vi "反控参数设置.vi"(8 "value time":timestamp, 9 "value float":sgl, 10 "设置参数":T2(ring)=enum."CODMn", 11 "设置类型":T1(ring)=enum."i13002") -> ()   [LabVIEW 2016, in "MB SLAVE.lvlib"]
uses:
  MB SLAVE.lvlib
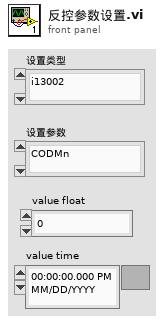
[diagram p1: front panel]
types:
  T1 = enum16{"i13001", "i13002", "i13003", "i13004", "i13005", "i13006", "i13007", "i13008", "i13009", "i13010", "i13011", "i13012", "i13013", "i13014", "i13015", "i13016", "i13017", "i13101", "i13102", "i13103", "i13104", "i13105", "i13106", "i13107", "i13108", "i13109", "i13110"}
  T2 = enum16{"", "CODMn", "PH", "氨氮", "总氮", "总磷", "CODCr", "电导率", "水温", "溶解氧", "浊度", "叶绿素", "藻密度", "ORP"}
  T3 = cluster{"status":bool, "代码":u16, "source":string}
  T4 = typedef "CODMn交互.ctl" = cluster{"COD浓度（mg/L)":dbl, "水样启动时间":timestamp, "加标回收启动时间":timestamp, "CODMn工作状态":enum16{"空闲", "水样测试", "标样核查", "零点核查", "跨度核查", "空白测试", "平行样测试", "加标回收", "空白校准", "标样校准", "初始化（清洗）"}, "多列列表框":i32, "平台试剂余量百分比":sgl, "关键参数":cluster{"测量量程":dbl, "测量精度":dbl, "测量间隔":dbl, "消解温度":dbl, "消解时长":dbl, "空白校准时间":timestamp, "曲线截距":dbl, "曲线斜率":dbl, "测量检出限":dbl, "测量信号值":dbl, "线性相关系数":dbl, "二次多项式系数":dbl, "标样校准时间":timestamp, "稀释倍数":dbl, "三项式系数":dbl, "空白标定系数":dbl, "量程系数":dbl, "F0/ORPA":dbl, "F1/ORPB":dbl, "F2/ORPK":dbl, "F3":dbl, "F4":dbl, "F5":dbl, "F6":dbl, "F7":dbl, "X0/滴定数":dbl, "量程":dbl}, "关键参数改变":bool, "校准信息":cluster{"低标液1浓度":dbl, "低标液1信号值":dbl, "低标液1启用":u16, "低标液2浓度":dbl, "低标液2信号值":dbl, "低标液2启用":u16, "低标液3浓度":dbl, "低标液3信号值":dbl, "低标液3启用":u16, "低标液4浓度":dbl, "低标液4信号值":dbl, "低标液4启用":u16, "低标液5浓度":dbl, "低标液5信号值":dbl, "低标液5启用":u16, "高标液1浓度":dbl, "高标液1信号值":dbl, "高标液1启用":u16, "高标液2浓度":dbl, "高标液2信号值":dbl, "高标液2启用":u16, "高标液3浓度":dbl, "高标液3信号值":dbl, "高标液3启用":u16, "高标液4浓度":dbl, "高标液4信号值":dbl, "高标液4启用":u16, "高标液5浓度":dbl, "高标液5信号值":dbl, "高标液5启用":u16}, "校准信息改变":bool}
  T5 = cluster{"测量量程":dbl, "测量精度":dbl, "测量间隔":dbl, "消解温度":dbl, "消解时长":dbl, "空白校准时间":timestamp, "曲线截距":dbl, "曲线斜率":dbl, "测量检出限":dbl, "测量信号值":dbl, "线性相关系数":dbl, "二次多项式系数":dbl, "标样校准时间":timestamp, "稀释倍数":dbl, "三项式系数":dbl, "空白标定系数":dbl, "量程系数":dbl, "F0/ORPA":dbl, "F1/ORPB":dbl, "F2/ORPK":dbl, "F3":dbl, "F4":dbl, "F5":dbl, "F6":dbl, "F7":dbl, "X0/滴定数":dbl, "量程":dbl}
  T6 = typedef "氨氮交互.ctl" = cluster{"状态告警区":cluster{"系统时间":timestamp, "工作状态":u16, "测量模式":enum16{"待机", "连续模式", "周期模式", "定点模式", "受控模式", "手动模式"}, "告警代码":u16, "故障代码":u16, "日志代码":u16, "软件版本":u16, "F0":sgl, "F1":sgl, "F2":sgl, "F3":sgl, "T":sgl, "H":sgl, "id":u16, "flowid":u16, "量程":u16, "总磷控温温度1":sgl, "营养盐控温温度2":sgl, "ADC":sgl}, "平台试剂余量百分比":sgl, "关键参数":cluster{"测量量程":dbl, "测量精度":dbl, "测量间隔":dbl, "消解温度":dbl, "消解时长":dbl, "空白校准时间":timestamp, "曲线截距":dbl, "曲线斜率":dbl, "测量检出限":dbl, "测量信号值":dbl, "线性相关系数":dbl, "二次多项式系数":dbl, "标样校准时间":timestamp, "稀释倍数":dbl, "三项式系数":dbl, "空白标定系数":dbl, "量程系数":dbl, "F0/ORPA":dbl, "F1/ORPB":dbl, "F2/ORPK":dbl, "F3":dbl, "F4":dbl, "F5":dbl, "F6":dbl, "F7":dbl, "X0/滴定数":dbl, "量程":dbl}, "关键参数改变":bool, "校准信息":cluster{"低标液1浓度":dbl, "低标液1信号值":dbl, "低标液1启用":u16, "低标液2浓度":dbl, "低标液2信号值":dbl, "低标液2启用":u16, "低标液3浓度":dbl, "低标液3信号值":dbl, "低标液3启用":u16, "低标液4浓度":dbl, "低标液4信号值":dbl, "低标液4启用":u16, "低标液5浓度":dbl, "低标液5信号值":dbl, "低标液5启用":u16, "高标液1浓度":dbl, "高标液1信号值":dbl, "高标液1启用":u16, "高标液2浓度":dbl, "高标液2信号值":dbl, "高标液2启用":u16, "高标液3浓度":dbl, "高标液3信号值":dbl, "高标液3启用":u16, "高标液4浓度":dbl, "高标液4信号值":dbl, "高标液4启用":u16, "高标液5浓度":dbl, "高标液5信号值":dbl, "高标液5启用":u16}, "校准信息改变":bool}
  T7 = typedef "总氮交互.ctl" = cluster{"状态告警区":cluster{"系统时间":timestamp, "工作状态":u16, "测量模式":enum16{"待机", "连续模式", "周期模式", "定点模式", "受控模式", "手动模式"}, "告警代码":u16, "故障代码":u16, "日志代码":u16, "软件版本":u16, "F0":sgl, "F1":sgl, "F2":sgl, "F3":sgl, "T":sgl, "H":sgl, "id":u16, "flowid":u16, "量程":u16, "总磷控温温度1":sgl, "营养盐控温温度2":sgl, "ADC":sgl}, "平台试剂余量百分比":sgl, "关键参数":cluster{"测量量程":dbl, "测量精度":dbl, "测量间隔":dbl, "消解温度":dbl, "消解时长":dbl, "空白校准时间":timestamp, "曲线截距":dbl, "曲线斜率":dbl, "测量检出限":dbl, "测量信号值":dbl, "线性相关系数":dbl, "二次多项式系数":dbl, "标样校准时间":timestamp, "稀释倍数":dbl, "三项式系数":dbl, "空白标定系数":dbl, "量程系数":dbl, "F0/ORPA":dbl, "F1/ORPB":dbl, "F2/ORPK":dbl, "F3":dbl, "F4":dbl, "F5":dbl, "F6":dbl, "F7":dbl, "X0/滴定数":dbl, "量程":dbl}, "关键参数改变":bool, "校准信息":cluster{"低标液1浓度":dbl, "低标液1信号值":dbl, "低标液1启用":u16, "低标液2浓度":dbl, "低标液2信号值":dbl, "低标液2启用":u16, "低标液3浓度":dbl, "低标液3信号值":dbl, "低标液3启用":u16, "低标液4浓度":dbl, "低标液4信号值":dbl, "低标液4启用":u16, "低标液5浓度":dbl, "低标液5信号值":dbl, "低标液5启用":u16, "高标液1浓度":dbl, "高标液1信号值":dbl, "高标液1启用":u16, "高标液2浓度":dbl, "高标液2信号值":dbl, "高标液2启用":u16, "高标液3浓度":dbl, "高标液3信号值":dbl, "高标液3启用":u16, "高标液4浓度":dbl, "高标液4信号值":dbl, "高标液4启用":u16, "高标液5浓度":dbl, "高标液5信号值":dbl, "高标液5启用":u16}, "校准信息改变":bool}
  T8 = typedef "总磷交互.ctl" = cluster{"状态告警区":cluster{"系统时间":timestamp, "工作状态":u16, "测量模式":enum16{"待机", "连续模式", "周期模式", "定点模式", "受控模式", "手动模式"}, "告警代码":u16, "故障代码":u16, "日志代码":u16, "软件版本":u16, "F0":sgl, "F1":sgl, "F2":sgl, "F3":sgl, "T":sgl, "H":sgl, "id":u16, "flowid":u16, "量程":u16, "总磷控温温度1":sgl, "营养盐控温温度2":sgl, "ADC":sgl}, "平台试剂余量百分比":sgl, "关键参数":cluster{"测量量程":dbl, "测量精度":dbl, "测量间隔":dbl, "消解温度":dbl, "消解时长":dbl, "空白校准时间":timestamp, "曲线截距":dbl, "曲线斜率":dbl, "测量检出限":dbl, "测量信号值":dbl, "线性相关系数":dbl, "二次多项式系数":dbl, "标样校准时间":timestamp, "稀释倍数":dbl, "三项式系数":dbl, "空白标定系数":dbl, "量程系数":dbl, "F0/ORPA":dbl, "F1/ORPB":dbl, "F2/ORPK":dbl, "F3":dbl, "F4":dbl, "F5":dbl, "F6":dbl, "F7":dbl, "X0/滴定数":dbl, "量程":dbl}, "关键参数改变":bool, "校准信息":cluster{"低标液1浓度":dbl, "低标液1信号值":dbl, "低标液1启用":u16, "低标液2浓度":dbl, "低标液2信号值":dbl, "低标液2启用":u16, "低标液3浓度":dbl, "低标液3信号值":dbl, "低标液3启用":u16, "低标液4浓度":dbl, "低标液4信号值":dbl, "低标液4启用":u16, "低标液5浓度":dbl, "低标液5信号值":dbl, "低标液5启用":u16, "高标液1浓度":dbl, "高标液1信号值":dbl, "高标液1启用":u16, "高标液2浓度":dbl, "高标液2信号值":dbl, "高标液2启用":u16, "高标液3浓度":dbl, "高标液3信号值":dbl, "高标液3启用":u16, "高标液4浓度":dbl, "高标液4信号值":dbl, "高标液4启用":u16, "高标液5浓度":dbl, "高标液5信号值":dbl, "高标液5启用":u16}, "校准信息改变":bool}
  T9 = typedef "CODCr交互.ctl" = cluster{"状态告警区":cluster{"系统时间":timestamp, "工作状态":u16, "测量模式":enum16{"待机", "连续模式", "周期模式", "定点模式", "受控模式", "手动模式"}, "告警代码":u16, "故障代码":u16, "日志代码":u16, "软件版本":u16, "F0":sgl, "F1":sgl, "F2":sgl, "F3":sgl, "T":sgl, "H":sgl, "id":u16, "flowid":u16, "量程":u16, "总磷控温温度1":sgl, "营养盐控温温度2":sgl, "ADC":sgl}, "平台试剂余量百分比":sgl, "关键参数":cluster{"测量量程":dbl, "测量精度":dbl, "测量间隔":dbl, "消解温度":dbl, "消解时长":dbl, "空白校准时间":timestamp, "曲线截距":dbl, "曲线斜率":dbl, "测量检出限":dbl, "测量信号值":dbl, "线性相关系数":dbl, "二次多项式系数":dbl, "标样校准时间":timestamp, "稀释倍数":dbl, "三项式系数":dbl, "空白标定系数":dbl, "量程系数":dbl, "F0/ORPA":dbl, "F1/ORPB":dbl, "F2/ORPK":dbl, "F3":dbl, "F4":dbl, "F5":dbl, "F6":dbl, "F7":dbl, "X0/滴定数":dbl, "量程":dbl}, "关键参数改变":bool, "校准信息":cluster{"低标液1浓度":dbl, "低标液1信号值":dbl, "低标液1启用":u16, "低标液2浓度":dbl, "低标液2信号值":dbl, "低标液2启用":u16, "低标液3浓度":dbl, "低标液3信号值":dbl, "低标液3启用":u16, "低标液4浓度":dbl, "低标液4信号值":dbl, "低标液4启用":u16, "低标液5浓度":dbl, "低标液5信号值":dbl, "低标液5启用":u16, "高标液1浓度":dbl, "高标液1信号值":dbl, "高标液1启用":u16, "高标液2浓度":dbl, "高标液2信号值":dbl, "高标液2启用":u16, "高标液3浓度":dbl, "高标液3信号值":dbl, "高标液3启用":u16, "高标液4浓度":dbl, "高标液4信号值":dbl, "高标液4启用":u16, "高标液5浓度":dbl, "高标液5信号值":dbl, "高标液5启用":u16}, "校准信息改变":bool}
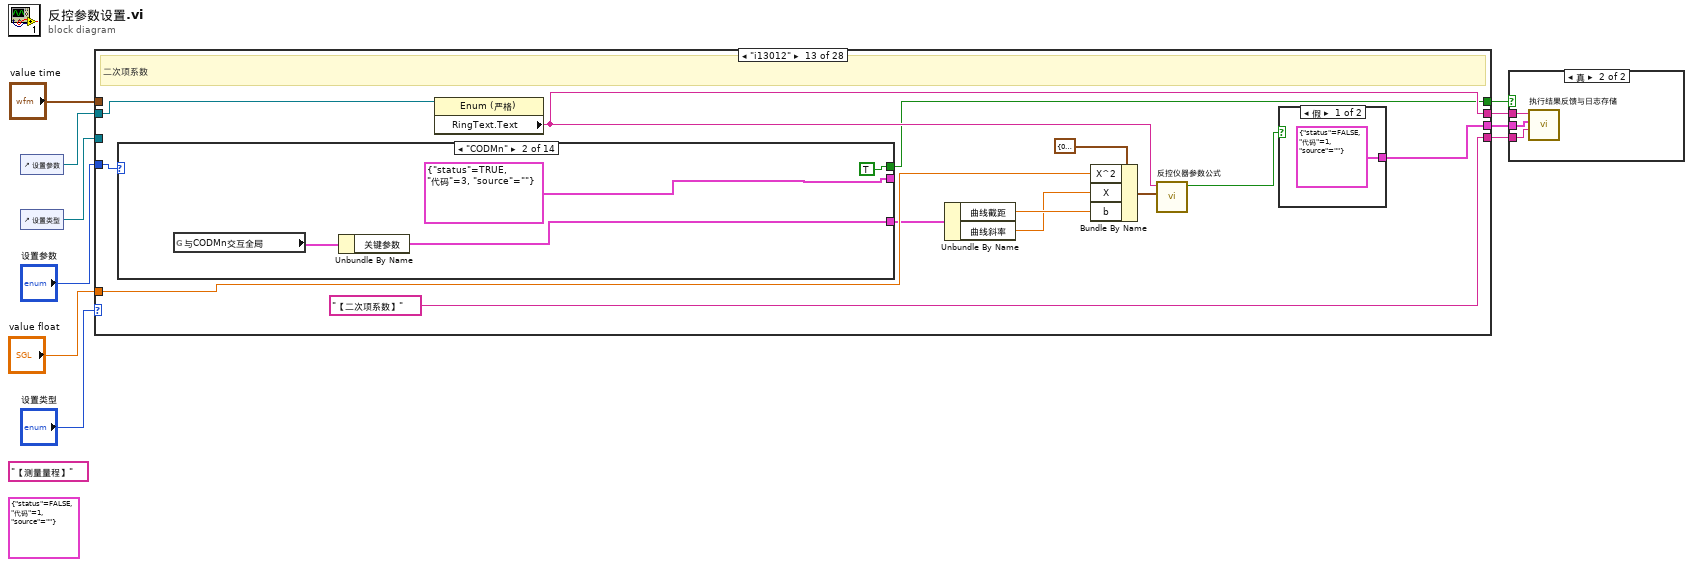
[diagram p0: block diagram]
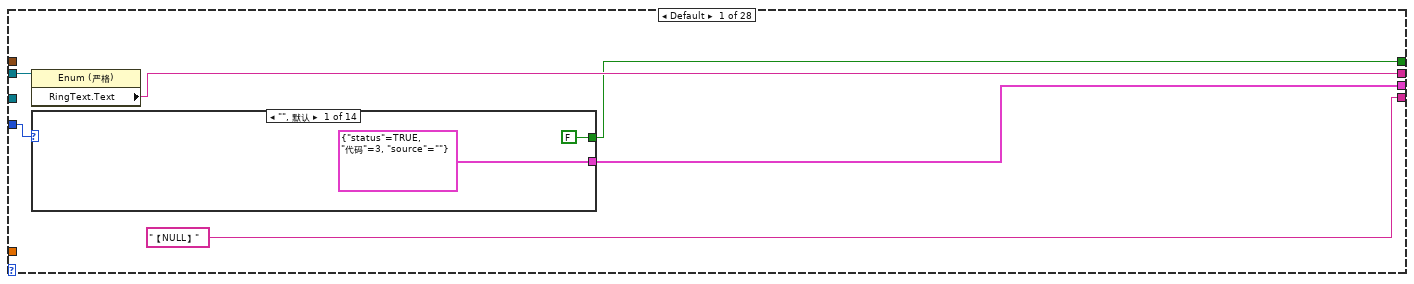
[diagram p3: hidden frame]
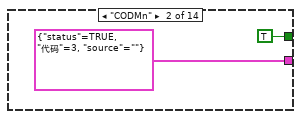
[diagram p4: hidden frame]
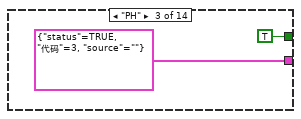
[diagram p5: hidden frame]
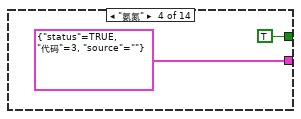
[diagram p6: hidden frame]
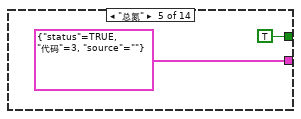
[diagram p7: hidden frame]
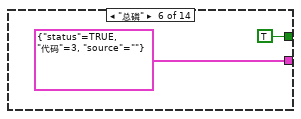
[diagram p8: hidden frame]
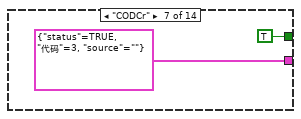
[diagram p9: hidden frame]
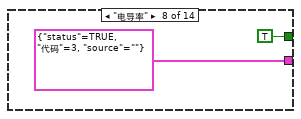
[diagram p10: hidden frame]
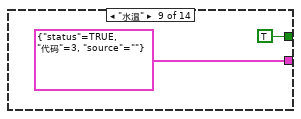
[diagram p11: hidden frame]
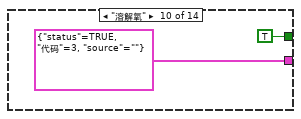
[diagram p12: hidden frame]
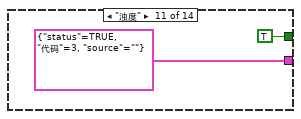
[diagram p13: hidden frame]
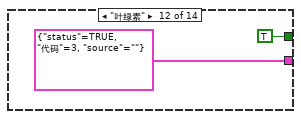
[diagram p14: hidden frame]
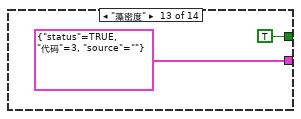
[diagram p15: hidden frame]
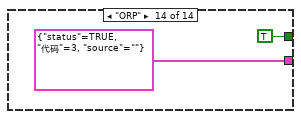
[diagram p16: hidden frame]
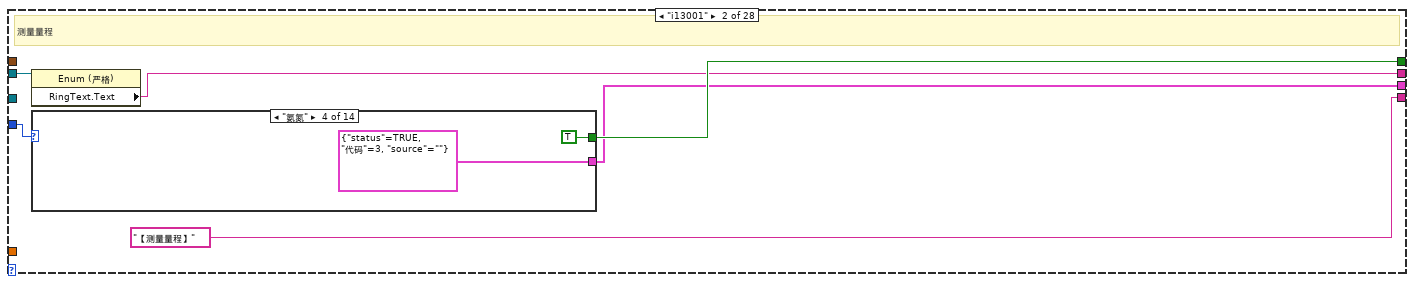
[diagram p17: hidden frame]
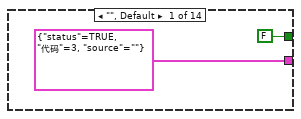
[diagram p18: hidden frame]
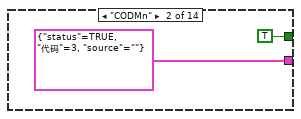
[diagram p19: hidden frame]
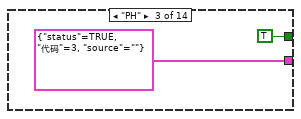
[diagram p20: hidden frame]
diagram:
  (unwired) T3 {"status"=FALSE, "代码"=1, "source"=""} ("error out")
  (unwired) "【测量量程】" ("日志信息")
  n1 = control-ref of="设置参数"() -> (w7:refnum<vi>)
  n2 = control-ref of="设置类型"() -> (w1:refnum<vi>)
  n3 = case shown="\"i13012\"" "设置类型" {
    tunnel: "设置参数" -> [w16 w50 w83 w114 w150 w193 w233 w269 w329 w373 w408 w444 w477 w528 w562 w596 w630 w664 w698 w732 w766 w804 w834 w868 w902 w936 w970 w1004]
    tunnel: [w12 w49 w80 w116 w152 w196 w236 w268 w332 w376 w410 w442 w476 w531 w565 w599 w633 w667 w701 w735 w769 w801 w837 w871 w905 w939 w973 w1007] -> w8
    tunnel: w7 -> [w15 w46 w84 w113 w154 w194 w234 w278 w330 w374 w407 w445 w486 w529 w563 w597 w631 w665 w699 w733 w767 w805 w835 w869 w903 w937 w971 w1005]
    tunnel: [w14 w45 w82 w118 w149 w190 w238 w274 w323 w378 w412 w446 w480 w533 w567 w601 w635 w669 w703 w737 w771 w803 w839 w873 w907 w941 w975 w1009] -> w6
    tunnel: ["【NULL】" ("日志信息") "【测量量程】" ("日志信息") "【测量精度】" ("日志信息") "【测量间隔】" ("日志信息") "【消解温度】" ("日志信息") "【消解时间】" ("日志信息") "【空白校准时间】" ("日志信息") "【曲线截距】" ("日志信息") "【曲线斜率】" ("日志信息") "【测量检出限】" ("日志信息") "【测量信号值】" ("日志信息") "【线性相关系数】" ("日志信息") "【二次项系数】" ("日志信息") "【标样校准时间】" ("日志信息") "【稀释倍数】" ("日志信息") "【三项式系数】" ("日志信息") "【空白标定系数】" ("日志信息") "【量程系数】" ("日志信息") "【F0/ORPA】" ("日志信息") "【F1/ORPB】" ("日志信息") "【F2/ORPK】" ("日志信息") "【F3】" ("日志信息") "【F4】" ("日志信息") "【F5】" ("日志信息") "【F6】" ("日志信息") "【F7】" ("日志信息") "【X0/滴定数】" ("日志信息") "【量程】" ("日志信息")] -> w5
    tunnel: [w13 w47 w81 w117 w153 w197 w237 w272 w325 w377 w411 w443 w482 w532 w566 w600 w634 w668 w702 w736 w770 w802 w838 w872 w906 w940 w974 w1008] -> w4
    tunnel: "value float" -> [_ _ _ _ w148 w192 _ w275 w324 _ _ _ w481 _ _ _ _ _ _ _ _ _ _ _ _ _ _ _]
    tunnel: "value time" -> [_ _ _ _ _ _ _ _ _ _ _ _ _ _ _ _ _ _ _ _ _ _ _ _ _ _ _ _]
    tunnel: w1 -> [_ _ _ _ w147 w191 _ _ _ _ _ _ _ _ _ _ _ _ _ _ _ _ _ _ _ _ _ _]
    frame Default {
      n4 = property class="Enum (严格)"(reference=w15) -> ("RingText.Text"=w14:string)  [unwired: 1 in, 2 out]
      n5 = case shown="\"\", 默认" w16 {
        tunnel: [FALSE TRUE TRUE TRUE TRUE TRUE TRUE TRUE TRUE TRUE TRUE TRUE TRUE TRUE] -> w12
        tunnel: [T3 {"status"=TRUE, "代码"=3, "source"=""} ("error out") T3 {"status"=TRUE, "代码"=3, "source"=""} ("error out") T3 {"status"=TRUE, "代码"=3, "source"=""} ("error out") T3 {"status"=TRUE, "代码"=3, "source"=""} ("error out") T3 {"status"=TRUE, "代码"=3, "source"=""} ("error out") T3 {"status"=TRUE, "代码"=3, "source"=""} ("error out") T3 {"status"=TRUE, "代码"=3, "source"=""} ("error out") T3 {"status"=TRUE, "代码"=3, "source"=""} ("error out") T3 {"status"=TRUE, "代码"=3, "source"=""} ("error out") T3 {"status"=TRUE, "代码"=3, "source"=""} ("error out") T3 {"status"=TRUE, "代码"=3, "source"=""} ("error out") T3 {"status"=TRUE, "代码"=3, "source"=""} ("error out") T3 {"status"=TRUE, "代码"=3, "source"=""} ("error out") T3 {"status"=TRUE, "代码"=3, "source"=""} ("error out")] -> w13
        frame "", Default {
        }
        frame "CODMn" {
        }
        frame "PH" {
        }
        frame "氨氮" {
        }
        frame "总氮" {
        }
        frame "总磷" {
        }
        frame "CODCr" {
        }
        frame "电导率" {
        }
        frame "水温" {
        }
        frame "溶解氧" {
        }
        frame "浊度" {
        }
        frame "叶绿素" {
        }
        frame "藻密度" {
        }
        frame "ORP" {
        }
      }
    }
    frame "i13001" {
      # "测量量程"
      n6 = property class="Enum (严格)"(reference=w46) -> ("RingText.Text"=w45:string)  [unwired: 1 in, 2 out]
      n7 = case shown="\"氨氮\"" w50 {
        tunnel: [FALSE TRUE TRUE TRUE TRUE TRUE TRUE TRUE TRUE TRUE TRUE TRUE TRUE TRUE] -> w49
        tunnel: [T3 {"status"=TRUE, "代码"=3, "source"=""} ("error out") T3 {"status"=TRUE, "代码"=3, "source"=""} ("error out") T3 {"status"=TRUE, "代码"=3, "source"=""} ("error out") T3 {"status"=TRUE, "代码"=3, "source"=""} ("error out") T3 {"status"=TRUE, "代码"=3, "source"=""} ("error out") T3 {"status"=TRUE, "代码"=3, "source"=""} ("error out") T3 {"status"=TRUE, "代码"=3, "source"=""} ("error out") T3 {"status"=TRUE, "代码"=3, "source"=""} ("error out") T3 {"status"=TRUE, "代码"=3, "source"=""} ("error out") T3 {"status"=TRUE, "代码"=3, "source"=""} ("error out") T3 {"status"=TRUE, "代码"=3, "source"=""} ("error out") T3 {"status"=TRUE, "代码"=3, "source"=""} ("error out") T3 {"status"=TRUE, "代码"=3, "source"=""} ("error out") T3 {"status"=TRUE, "代码"=3, "source"=""} ("error out")] -> w47
        frame "", Default {
        }
        frame "CODMn" {
        }
        frame "PH" {
        }
        frame "氨氮" {
        }
        frame "总氮" {
        }
        frame "总磷" {
        }
        frame "CODCr" {
        }
        frame "电导率" {
        }
        frame "水温" {
        }
        frame "溶解氧" {
        }
        frame "浊度" {
        }
        frame "叶绿素" {
        }
        frame "藻密度" {
        }
        frame "ORP" {
        }
      }
    }
    frame "i13002" {
      # "测量精度"
      n8 = property class="Enum (严格)"(reference=w84) -> ("RingText.Text"=w82:string)  [unwired: 1 in, 2 out]
      n9 = case shown="\"CODMn\"" w83 {
        tunnel: [FALSE TRUE TRUE TRUE TRUE TRUE TRUE TRUE TRUE TRUE TRUE TRUE TRUE TRUE] -> w80
        tunnel: [T3 {"status"=TRUE, "代码"=3, "source"=""} ("error out") T3 {"status"=TRUE, "代码"=3, "source"=""} ("error out") T3 {"status"=TRUE, "代码"=3, "source"=""} ("error out") T3 {"status"=TRUE, "代码"=3, "source"=""} ("error out") T3 {"status"=TRUE, "代码"=3, "source"=""} ("error out") T3 {"status"=TRUE, "代码"=3, "source"=""} ("error out") T3 {"status"=TRUE, "代码"=3, "source"=""} ("error out") T3 {"status"=TRUE, "代码"=3, "source"=""} ("error out") T3 {"status"=TRUE, "代码"=3, "source"=""} ("error out") T3 {"status"=TRUE, "代码"=3, "source"=""} ("error out") T3 {"status"=TRUE, "代码"=3, "source"=""} ("error out") T3 {"status"=TRUE, "代码"=3, "source"=""} ("error out") T3 {"status"=TRUE, "代码"=3, "source"=""} ("error out") T3 {"status"=TRUE, "代码"=3, "source"=""} ("error out")] -> w81
        frame "", Default {
        }
        frame "CODMn" {
        }
        frame "PH" {
        }
        frame "氨氮" {
        }
        frame "总氮" {
        }
        frame "总磷" {
        }
        frame "CODCr" {
        }
        frame "电导率" {
        }
        frame "水温" {
        }
        frame "溶解氧" {
        }
        frame "浊度" {
        }
        frame "叶绿素" {
        }
        frame "藻密度" {
        }
        frame "ORP" {
        }
      }
    }
    frame "i13003" {
      # "测量间隔"
      n10 = property class="Enum (严格)"(reference=w113) -> ("RingText.Text"=w118:string)  [unwired: 1 in, 2 out]
      n11 = case shown="\"CODMn\"" w114 {
        tunnel: [FALSE TRUE TRUE TRUE TRUE TRUE TRUE TRUE TRUE TRUE TRUE TRUE TRUE TRUE] -> w116
        tunnel: [T3 {"status"=TRUE, "代码"=3, "source"=""} ("error out") T3 {"status"=TRUE, "代码"=3, "source"=""} ("error out") T3 {"status"=TRUE, "代码"=3, "source"=""} ("error out") T3 {"status"=TRUE, "代码"=3, "source"=""} ("error out") T3 {"status"=TRUE, "代码"=3, "source"=""} ("error out") T3 {"status"=TRUE, "代码"=3, "source"=""} ("error out") T3 {"status"=TRUE, "代码"=3, "source"=""} ("error out") T3 {"status"=TRUE, "代码"=3, "source"=""} ("error out") T3 {"status"=TRUE, "代码"=3, "source"=""} ("error out") T3 {"status"=TRUE, "代码"=3, "source"=""} ("error out") T3 {"status"=TRUE, "代码"=3, "source"=""} ("error out") T3 {"status"=TRUE, "代码"=3, "source"=""} ("error out") T3 {"status"=TRUE, "代码"=3, "source"=""} ("error out") T3 {"status"=TRUE, "代码"=3, "source"=""} ("error out")] -> w117
        frame "", Default {
        }
        frame "CODMn" {
        }
        frame "PH" {
        }
        frame "氨氮" {
        }
        frame "总氮" {
        }
        frame "总磷" {
        }
        frame "CODCr" {
        }
        frame "电导率" {
        }
        frame "水温" {
        }
        frame "溶解氧" {
        }
        frame "浊度" {
        }
        frame "叶绿素" {
        }
        frame "藻密度" {
        }
        frame "ORP" {
        }
      }
    }
    frame "i13004" {
      # "消解温度"
      n12 = property class="Enum (严格)"(reference=w154) -> ("RingText.Text"=w149:string)  [unwired: 1 in, 2 out]
      n13 = case shown="\"氨氮\"" w150 {
        tunnel: [FALSE TRUE TRUE TRUE TRUE TRUE TRUE TRUE TRUE TRUE TRUE TRUE TRUE TRUE] -> w152
        tunnel: [T3 {"status"=TRUE, "代码"=3, "source"=""} ("error out") w159 T3 {"status"=TRUE, "代码"=3, "source"=""} ("error out") T3 {"status"=TRUE, "代码"=3, "source"=""} ("error out") T3 {"status"=TRUE, "代码"=3, "source"=""} ("error out") T3 {"status"=TRUE, "代码"=3, "source"=""} ("error out") T3 {"status"=TRUE, "代码"=3, "source"=""} ("error out") T3 {"status"=TRUE, "代码"=3, "source"=""} ("error out") T3 {"status"=TRUE, "代码"=3, "source"=""} ("error out") T3 {"status"=TRUE, "代码"=3, "source"=""} ("error out") T3 {"status"=TRUE, "代码"=3, "source"=""} ("error out") T3 {"status"=TRUE, "代码"=3, "source"=""} ("error out") T3 {"status"=TRUE, "代码"=3, "source"=""} ("error out") T3 {"status"=TRUE, "代码"=3, "source"=""} ("error out")] -> w153
        tunnel: w149 -> [_ w162 _ _ _ _ _ _ _ _ _ _ _ _]
        tunnel: w148 -> [_ w161 _ _ _ _ _ _ _ _ _ _ _ _]
        tunnel: w147 -> [_ w158 _ _ _ _ _ _ _ _ _ _ _ _]
        frame "", Default {
        }
        frame "CODMn" {
          n14 = property class="Enum (严格)"(reference=w158) -> ("RingText.Text"=w157:string)  [unwired: 1 in, 2 out]
          n15 = call "反控仪器单参数通用.vi"("参数"=w162, "value float"=w161, "chose"=w157) -> ("超时？"=w160:bool)  [unwired: 7 in, 1 out]
          n16 = case shown="假" w160 {
            tunnel: [T3 {"status"=FALSE, "代码"=1, "source"=""} ("error out") T3 {"status"=TRUE, "代码"=4, "source"=""} ("error out")] -> w159
            frame False {
            }
            frame True {
            }
          }
        }
        frame "PH" {
        }
        frame "氨氮" {
        }
        frame "总氮" {
        }
        frame "总磷" {
        }
        frame "CODCr" {
        }
        frame "电导率" {
        }
        frame "水温" {
        }
        frame "溶解氧" {
        }
        frame "浊度" {
        }
        frame "叶绿素" {
        }
        frame "藻密度" {
        }
        frame "ORP" {
        }
      }
    }
    frame "i13005" {
      # "消解时间"
      n17 = property class="Enum (严格)"(reference=w194) -> ("RingText.Text"=w190:string)  [unwired: 1 in, 2 out]
      n18 = case shown="\"CODMn\"" w193 {
        tunnel: [FALSE TRUE TRUE TRUE TRUE TRUE TRUE TRUE TRUE TRUE TRUE TRUE TRUE TRUE] -> w196
        tunnel: [T3 {"status"=TRUE, "代码"=3, "source"=""} ("error out") w200 T3 {"status"=TRUE, "代码"=3, "source"=""} ("error out") T3 {"status"=TRUE, "代码"=3, "source"=""} ("error out") T3 {"status"=TRUE, "代码"=3, "source"=""} ("error out") T3 {"status"=TRUE, "代码"=3, "source"=""} ("error out") T3 {"status"=TRUE, "代码"=3, "source"=""} ("error out") T3 {"status"=TRUE, "代码"=3, "source"=""} ("error out") T3 {"status"=TRUE, "代码"=3, "source"=""} ("error out") T3 {"status"=TRUE, "代码"=3, "source"=""} ("error out") T3 {"status"=TRUE, "代码"=3, "source"=""} ("error out") T3 {"status"=TRUE, "代码"=3, "source"=""} ("error out") T3 {"status"=TRUE, "代码"=3, "source"=""} ("error out") T3 {"status"=TRUE, "代码"=3, "source"=""} ("error out")] -> w197
        tunnel: w192 -> [_ w203 _ _ _ _ _ _ _ _ _ _ _ _]
        tunnel: w191 -> [_ w202 _ _ _ _ _ _ _ _ _ _ _ _]
        tunnel: w190 -> [_ w201 _ _ _ _ _ _ _ _ _ _ _ _]
        frame "", Default {
        }
        frame "CODMn" {
          n19 = property class="Enum (严格)"(reference=w202) -> ("RingText.Text"=w204:string)  [unwired: 1 in, 2 out]
          n20 = call "反控仪器单参数通用.vi"("参数"=w201, "value float"=w203, "chose"=w204) -> ("超时？"=w205:bool)  [unwired: 7 in, 1 out]
          n21 = case shown="假" w205 {
            tunnel: [T3 {"status"=FALSE, "代码"=1, "source"=""} ("error out") T3 {"status"=TRUE, "代码"=4, "source"=""} ("error out")] -> w200
            frame False {
            }
            frame True {
            }
          }
        }
        frame "PH" {
        }
        frame "氨氮" {
        }
        frame "总氮" {
        }
        frame "总磷" {
        }
        frame "CODCr" {
        }
        frame "电导率" {
        }
        frame "水温" {
        }
        frame "溶解氧" {
        }
        frame "浊度" {
        }
        frame "叶绿素" {
        }
        frame "藻密度" {
        }
        frame "ORP" {
        }
      }
    }
    frame "i13006" {
      # "空白校准时间"
      n22 = property class="Enum (严格)"(reference=w234) -> ("RingText.Text"=w238:string)  [unwired: 1 in, 2 out]
      n23 = case shown="\"CODMn\"" w233 {
        tunnel: [FALSE TRUE TRUE TRUE TRUE TRUE TRUE TRUE TRUE TRUE TRUE TRUE TRUE TRUE] -> w236
        tunnel: [T3 {"status"=TRUE, "代码"=3, "source"=""} ("error out") T3 {"status"=TRUE, "代码"=3, "source"=""} ("error out") T3 {"status"=TRUE, "代码"=3, "source"=""} ("error out") T3 {"status"=TRUE, "代码"=3, "source"=""} ("error out") T3 {"status"=TRUE, "代码"=3, "source"=""} ("error out") T3 {"status"=TRUE, "代码"=3, "source"=""} ("error out") T3 {"status"=TRUE, "代码"=3, "source"=""} ("error out") T3 {"status"=TRUE, "代码"=3, "source"=""} ("error out") T3 {"status"=TRUE, "代码"=3, "source"=""} ("error out") T3 {"status"=TRUE, "代码"=3, "source"=""} ("error out") T3 {"status"=TRUE, "代码"=3, "source"=""} ("error out") T3 {"status"=TRUE, "代码"=3, "source"=""} ("error out") T3 {"status"=TRUE, "代码"=3, "source"=""} ("error out") T3 {"status"=TRUE, "代码"=3, "source"=""} ("error out")] -> w237
        frame "", Default {
        }
        frame "CODMn" {
        }
        frame "PH" {
        }
        frame "氨氮" {
        }
        frame "总氮" {
        }
        frame "总磷" {
        }
        frame "CODCr" {
        }
        frame "电导率" {
        }
        frame "水温" {
        }
        frame "溶解氧" {
        }
        frame "浊度" {
        }
        frame "叶绿素" {
        }
        frame "藻密度" {
        }
        frame "ORP" {
        }
      }
    }
    frame "i13007" {
      # "曲线截距"
      n24 = case shown="\"CODMn\"" w269 {
        tunnel: [FALSE TRUE TRUE TRUE TRUE TRUE TRUE TRUE TRUE TRUE TRUE TRUE TRUE TRUE] -> w268
        tunnel: [T3 {"status"=TRUE, "代码"=3, "source"=""} ("error out") T3 {"status"=TRUE, "代码"=3, "source"=""} ("error out") T3 {"status"=TRUE, "代码"=3, "source"=""} ("error out") T3 {"status"=TRUE, "代码"=3, "source"=""} ("error out") T3 {"status"=TRUE, "代码"=3, "source"=""} ("error out") T3 {"status"=TRUE, "代码"=3, "source"=""} ("error out") T3 {"status"=TRUE, "代码"=3, "source"=""} ("error out") T3 {"status"=TRUE, "代码"=3, "source"=""} ("error out") T3 {"status"=TRUE, "代码"=3, "source"=""} ("error out") T3 {"status"=TRUE, "代码"=3, "source"=""} ("error out") T3 {"status"=TRUE, "代码"=3, "source"=""} ("error out") T3 {"status"=TRUE, "代码"=3, "source"=""} ("error out") T3 {"status"=TRUE, "代码"=3, "source"=""} ("error out") T3 {"status"=TRUE, "代码"=3, "source"=""} ("error out")] -> _
        tunnel: [_ w282 _ w288 w292 w296 w300 _ _ _ _ _ _ _] -> w267
        frame "", Default {
        }
        frame "CODMn" {
          n25 = global read "modbus slave全局.vi" "与CODMn交互全局"() -> (w283:T4)
          n26 = Unbundle By Name(w283) -> ("关键参数"=w282:T5)
        }
        frame "PH" {
        }
        frame "氨氮" {
          n27 = global read "modbus slave全局.vi" "与氨氮交互全局"() -> (w289:T6)
          n28 = Unbundle By Name(w289) -> ("关键参数"=w288:T5)
        }
        frame "总氮" {
          n29 = global read "modbus slave全局.vi" "与总氮交互全局"() -> (w293:T7)
          n30 = Unbundle By Name(w293) -> ("关键参数"=w292:T5)
        }
        frame "总磷" {
          n31 = global read "modbus slave全局.vi" "与总磷交互全局"() -> (w297:T8)
          n32 = Unbundle By Name(w297) -> ("关键参数"=w296:T5)
        }
        frame "CODCr" {
          n33 = global read "modbus slave全局.vi" "与CODCr交互全局"() -> (w301:T9)
          n34 = Unbundle By Name(w301) -> ("关键参数"=w300:T5)
        }
        frame "电导率" {
        }
        frame "水温" {
        }
        frame "溶解氧" {
        }
        frame "浊度" {
        }
        frame "叶绿素" {
        }
        frame "藻密度" {
        }
        frame "ORP" {
        }
      }
      n35 = property class="Enum (严格)"(reference=w278) -> ("RingText.Text"=w274:string)  [unwired: 1 in, 2 out]
      n36 = Unbundle By Name(w267) -> ("曲线斜率"=w271:dbl, "二次多项式系数"=w270:dbl)
      n37 = Bundle By Name(cluster=cluster{"X^2":dbl, "X":dbl, "b":dbl} {"X^2"=0.0, "X"=0.0, "b"=0.0} ("公式"), "X^2"=w270, "X"=w271, "b"=w275) -> (w277:cluster{"X^2":dbl, "X":dbl, "b":dbl})
      n38 = call "反控仪器参数公式.vi"("公式"=w277, "参数"=w274) -> ("超时？"=w273:bool)  [unwired: 8 in, 1 out]
      n39 = case shown="假" w273 {
        tunnel: [T3 {"status"=FALSE, "代码"=1, "source"=""} ("error out") T3 {"status"=TRUE, "代码"=4, "source"=""} ("error out")] -> w272
        frame False {
        }
        frame True {
        }
      }
    }
    frame "i13008" {
      # "曲线斜率"
      n40 = case shown="\"CODMn\"" w329 {
        tunnel: [FALSE TRUE TRUE TRUE TRUE TRUE TRUE TRUE TRUE TRUE TRUE TRUE TRUE TRUE] -> w332
        tunnel: [T3 {"status"=TRUE, "代码"=3, "source"=""} ("error out") T3 {"status"=TRUE, "代码"=3, "source"=""} ("error out") T3 {"status"=TRUE, "代码"=3, "source"=""} ("error out") T3 {"status"=TRUE, "代码"=3, "source"=""} ("error out") T3 {"status"=TRUE, "代码"=3, "source"=""} ("error out") T3 {"status"=TRUE, "代码"=3, "source"=""} ("error out") T3 {"status"=TRUE, "代码"=3, "source"=""} ("error out") T3 {"status"=TRUE, "代码"=3, "source"=""} ("error out") T3 {"status"=TRUE, "代码"=3, "source"=""} ("error out") T3 {"status"=TRUE, "代码"=3, "source"=""} ("error out") T3 {"status"=TRUE, "代码"=3, "source"=""} ("error out") T3 {"status"=TRUE, "代码"=3, "source"=""} ("error out") T3 {"status"=TRUE, "代码"=3, "source"=""} ("error out") T3 {"status"=TRUE, "代码"=3, "source"=""} ("error out")] -> _
        tunnel: [_ w337 _ w343 w347 w351 w355 _ _ _ _ _ _ _] -> w320
        frame "", Default {
        }
        frame "CODMn" {
          n41 = global read "modbus slave全局.vi" "与CODMn交互全局"() -> (w338:T4)
          n42 = Unbundle By Name(w338) -> ("关键参数"=w337:T5)
        }
        frame "PH" {
        }
        frame "氨氮" {
          n43 = global read "modbus slave全局.vi" "与氨氮交互全局"() -> (w344:T6)
          n44 = Unbundle By Name(w344) -> ("关键参数"=w343:T5)
        }
        frame "总氮" {
          n45 = global read "modbus slave全局.vi" "与总氮交互全局"() -> (w348:T7)
          n46 = Unbundle By Name(w348) -> ("关键参数"=w347:T5)
        }
        frame "总磷" {
          n47 = global read "modbus slave全局.vi" "与总磷交互全局"() -> (w352:T8)
          n48 = Unbundle By Name(w352) -> ("关键参数"=w351:T5)
        }
        frame "CODCr" {
          n49 = global read "modbus slave全局.vi" "与CODCr交互全局"() -> (w356:T9)
          n50 = Unbundle By Name(w356) -> ("关键参数"=w355:T5)
        }
        frame "电导率" {
        }
        frame "水温" {
        }
        frame "溶解氧" {
        }
        frame "浊度" {
        }
        frame "叶绿素" {
        }
        frame "藻密度" {
        }
        frame "ORP" {
        }
      }
      n51 = property class="Enum (严格)"(reference=w330) -> ("RingText.Text"=w323:string)  [unwired: 1 in, 2 out]
      n52 = Unbundle By Name(w320) -> ("曲线截距"=w321:dbl, "二次多项式系数"=w322:dbl)
      n53 = Bundle By Name(cluster=cluster{"X^2":dbl, "X":dbl, "b":dbl} {"X^2"=0.0, "X"=0.0, "b"=0.0} ("公式"), "X^2"=w322, "X"=w324, "b"=w321) -> (w326:cluster{"X^2":dbl, "X":dbl, "b":dbl})
      n54 = call "反控仪器参数公式.vi"("公式"=w326, "参数"=w323) -> ("超时？"=w328:bool)  [unwired: 8 in, 1 out]
      n55 = case shown="假" w328 {
        tunnel: [T3 {"status"=FALSE, "代码"=1, "source"=""} ("error out") T3 {"status"=TRUE, "代码"=4, "source"=""} ("error out")] -> w325
        frame False {
        }
        frame True {
        }
      }
    }
    frame "i13009" {
      # "测量检出限"
      n56 = property class="Enum (严格)"(reference=w374) -> ("RingText.Text"=w378:string)  [unwired: 1 in, 2 out]
      n57 = case shown="\"PH\"" w373 {
        tunnel: [FALSE TRUE TRUE TRUE TRUE TRUE TRUE TRUE TRUE TRUE TRUE TRUE TRUE TRUE] -> w376
        tunnel: [T3 {"status"=TRUE, "代码"=3, "source"=""} ("error out") T3 {"status"=TRUE, "代码"=3, "source"=""} ("error out") T3 {"status"=TRUE, "代码"=3, "source"=""} ("error out") T3 {"status"=TRUE, "代码"=3, "source"=""} ("error out") T3 {"status"=TRUE, "代码"=3, "source"=""} ("error out") T3 {"status"=TRUE, "代码"=3, "source"=""} ("error out") T3 {"status"=TRUE, "代码"=3, "source"=""} ("error out") T3 {"status"=TRUE, "代码"=3, "source"=""} ("error out") T3 {"status"=TRUE, "代码"=3, "source"=""} ("error out") T3 {"status"=TRUE, "代码"=3, "source"=""} ("error out") T3 {"status"=TRUE, "代码"=3, "source"=""} ("error out") T3 {"status"=TRUE, "代码"=3, "source"=""} ("error out") T3 {"status"=TRUE, "代码"=3, "source"=""} ("error out") T3 {"status"=TRUE, "代码"=3, "source"=""} ("error out")] -> w377
        frame "", Default {
        }
        frame "CODMn" {
        }
        frame "PH" {
        }
        frame "氨氮" {
        }
        frame "总氮" {
        }
        frame "总磷" {
        }
        frame "CODCr" {
        }
        frame "电导率" {
        }
        frame "水温" {
        }
        frame "溶解氧" {
        }
        frame "浊度" {
        }
        frame "叶绿素" {
        }
        frame "藻密度" {
        }
        frame "ORP" {
        }
      }
    }
    frame "i13010" {
      # "测量信号值"
      n58 = property class="Enum (严格)"(reference=w407) -> ("RingText.Text"=w412:string)  [unwired: 1 in, 2 out]
      n59 = case shown="\"PH\"" w408 {
        tunnel: [FALSE TRUE TRUE TRUE TRUE TRUE TRUE TRUE TRUE TRUE TRUE TRUE TRUE TRUE] -> w410
        tunnel: [T3 {"status"=TRUE, "代码"=3, "source"=""} ("error out") T3 {"status"=TRUE, "代码"=3, "source"=""} ("error out") T3 {"status"=TRUE, "代码"=3, "source"=""} ("error out") T3 {"status"=TRUE, "代码"=3, "source"=""} ("error out") T3 {"status"=TRUE, "代码"=3, "source"=""} ("error out") T3 {"status"=TRUE, "代码"=3, "source"=""} ("error out") T3 {"status"=TRUE, "代码"=3, "source"=""} ("error out") T3 {"status"=TRUE, "代码"=3, "source"=""} ("error out") T3 {"status"=TRUE, "代码"=3, "source"=""} ("error out") T3 {"status"=TRUE, "代码"=3, "source"=""} ("error out") T3 {"status"=TRUE, "代码"=3, "source"=""} ("error out") T3 {"status"=TRUE, "代码"=3, "source"=""} ("error out") T3 {"status"=TRUE, "代码"=3, "source"=""} ("error out") T3 {"status"=TRUE, "代码"=3, "source"=""} ("error out")] -> w411
        frame "", Default {
        }
        frame "CODMn" {
        }
        frame "PH" {
        }
        frame "氨氮" {
        }
        frame "总氮" {
        }
        frame "总磷" {
        }
        frame "CODCr" {
        }
        frame "电导率" {
        }
        frame "水温" {
        }
        frame "溶解氧" {
        }
        frame "浊度" {
        }
        frame "叶绿素" {
        }
        frame "藻密度" {
        }
        frame "ORP" {
        }
      }
    }
    frame "i13011" {
      # "线性相关系数"
      n60 = property class="Enum (严格)"(reference=w445) -> ("RingText.Text"=w446:string)  [unwired: 1 in, 2 out]
      n61 = case shown="\"氨氮\"" w444 {
        tunnel: [FALSE TRUE TRUE TRUE TRUE TRUE TRUE TRUE TRUE TRUE TRUE TRUE TRUE TRUE] -> w442
        tunnel: [T3 {"status"=TRUE, "代码"=3, "source"=""} ("error out") T3 {"status"=TRUE, "代码"=3, "source"=""} ("error out") T3 {"status"=TRUE, "代码"=3, "source"=""} ("error out") T3 {"status"=TRUE, "代码"=3, "source"=""} ("error out") T3 {"status"=TRUE, "代码"=3, "source"=""} ("error out") T3 {"status"=TRUE, "代码"=3, "source"=""} ("error out") T3 {"status"=TRUE, "代码"=3, "source"=""} ("error out") T3 {"status"=TRUE, "代码"=3, "source"=""} ("error out") T3 {"status"=TRUE, "代码"=3, "source"=""} ("error out") T3 {"status"=TRUE, "代码"=3, "source"=""} ("error out") T3 {"status"=TRUE, "代码"=3, "source"=""} ("error out") T3 {"status"=TRUE, "代码"=3, "source"=""} ("error out") T3 {"status"=TRUE, "代码"=3, "source"=""} ("error out") T3 {"status"=TRUE, "代码"=3, "source"=""} ("error out")] -> w443
        frame "", Default {
        }
        frame "CODMn" {
        }
        frame "PH" {
        }
        frame "氨氮" {
        }
        frame "总氮" {
        }
        frame "总磷" {
        }
        frame "CODCr" {
        }
        frame "电导率" {
        }
        frame "水温" {
        }
        frame "溶解氧" {
        }
        frame "浊度" {
        }
        frame "叶绿素" {
        }
        frame "藻密度" {
        }
        frame "ORP" {
        }
      }
    }
    frame "i13012" {
      # "二次项系数"
      n62 = case shown="\"CODMn\"" w477 {
        tunnel: [FALSE TRUE TRUE TRUE TRUE TRUE TRUE TRUE TRUE TRUE TRUE TRUE TRUE TRUE] -> w476
        tunnel: [T3 {"status"=TRUE, "代码"=3, "source"=""} ("error out") T3 {"status"=TRUE, "代码"=3, "source"=""} ("error out") T3 {"status"=TRUE, "代码"=3, "source"=""} ("error out") T3 {"status"=TRUE, "代码"=3, "source"=""} ("error out") T3 {"status"=TRUE, "代码"=3, "source"=""} ("error out") T3 {"status"=TRUE, "代码"=3, "source"=""} ("error out") T3 {"status"=TRUE, "代码"=3, "source"=""} ("error out") T3 {"status"=TRUE, "代码"=3, "source"=""} ("error out") T3 {"status"=TRUE, "代码"=3, "source"=""} ("error out") T3 {"status"=TRUE, "代码"=3, "source"=""} ("error out") T3 {"status"=TRUE, "代码"=3, "source"=""} ("error out") T3 {"status"=TRUE, "代码"=3, "source"=""} ("error out") T3 {"status"=TRUE, "代码"=3, "source"=""} ("error out") T3 {"status"=TRUE, "代码"=3, "source"=""} ("error out")] -> _
        tunnel: [_ w490 _ w496 w500 w504 w508 _ _ _ _ _ _ _] -> w475
        frame "", Default {
        }
        frame "CODMn" {
          n63 = global read "modbus slave全局.vi" "与CODMn交互全局"() -> (w491:T4)
          n64 = Unbundle By Name(w491) -> ("关键参数"=w490:T5)
        }
        frame "PH" {
        }
        frame "氨氮" {
          n65 = global read "modbus slave全局.vi" "与氨氮交互全局"() -> (w497:T6)
          n66 = Unbundle By Name(w497) -> ("关键参数"=w496:T5)
        }
        frame "总氮" {
          n67 = global read "modbus slave全局.vi" "与总氮交互全局"() -> (w501:T7)
          n68 = Unbundle By Name(w501) -> ("关键参数"=w500:T5)
        }
        frame "总磷" {
          n69 = global read "modbus slave全局.vi" "与总磷交互全局"() -> (w505:T8)
          n70 = Unbundle By Name(w505) -> ("关键参数"=w504:T5)
        }
        frame "CODCr" {
          n71 = global read "modbus slave全局.vi" "与CODCr交互全局"() -> (w509:T9)
          n72 = Unbundle By Name(w509) -> ("关键参数"=w508:T5)
        }
        frame "电导率" {
        }
        frame "水温" {
        }
        frame "溶解氧" {
        }
        frame "浊度" {
        }
        frame "叶绿素" {
        }
        frame "藻密度" {
        }
        frame "ORP" {
        }
      }
      n73 = property class="Enum (严格)"(reference=w486) -> ("RingText.Text"=w480:string)  [unwired: 1 in, 2 out]
      n74 = Unbundle By Name(w475) -> ("曲线截距"=w479:dbl, "曲线斜率"=w478:dbl)
      n75 = Bundle By Name(cluster=cluster{"X^2":dbl, "X":dbl, "b":dbl} {"X^2"=0.0, "X"=0.0, "b"=0.0} ("公式"), "X^2"=w481, "X"=w478, "b"=w479) -> (w483:cluster{"X^2":dbl, "X":dbl, "b":dbl})
      n76 = call "反控仪器参数公式.vi"("公式"=w483, "参数"=w480) -> ("超时？"=w485:bool)  [unwired: 8 in, 1 out]
      n77 = case shown="假" w485 {
        tunnel: [T3 {"status"=FALSE, "代码"=1, "source"=""} ("error out") T3 {"status"=TRUE, "代码"=4, "source"=""} ("error out")] -> w482
        frame False {
        }
        frame True {
        }
      }
    }
    frame "i13013" {
      # "标样校准时间"
      n78 = property class="Enum (严格)"(reference=w529) -> ("RingText.Text"=w533:string)  [unwired: 1 in, 2 out]
      n79 = case shown="\"CODMn\"" w528 {
        tunnel: [FALSE TRUE TRUE TRUE TRUE TRUE TRUE TRUE TRUE TRUE TRUE TRUE TRUE TRUE] -> w531
        tunnel: [T3 {"status"=TRUE, "代码"=3, "source"=""} ("error out") T3 {"status"=TRUE, "代码"=3, "source"=""} ("error out") T3 {"status"=TRUE, "代码"=3, "source"=""} ("error out") T3 {"status"=TRUE, "代码"=3, "source"=""} ("error out") T3 {"status"=TRUE, "代码"=3, "source"=""} ("error out") T3 {"status"=TRUE, "代码"=3, "source"=""} ("error out") T3 {"status"=TRUE, "代码"=3, "source"=""} ("error out") T3 {"status"=TRUE, "代码"=3, "source"=""} ("error out") T3 {"status"=TRUE, "代码"=3, "source"=""} ("error out") T3 {"status"=TRUE, "代码"=3, "source"=""} ("error out") T3 {"status"=TRUE, "代码"=3, "source"=""} ("error out") T3 {"status"=TRUE, "代码"=3, "source"=""} ("error out") T3 {"status"=TRUE, "代码"=3, "source"=""} ("error out") T3 {"status"=TRUE, "代码"=3, "source"=""} ("error out")] -> w532
        frame "", Default {
        }
        frame "CODMn" {
        }
        frame "PH" {
        }
        frame "氨氮" {
        }
        frame "总氮" {
        }
        frame "总磷" {
        }
        frame "CODCr" {
        }
        frame "电导率" {
        }
        frame "水温" {
        }
        frame "溶解氧" {
        }
        frame "浊度" {
        }
        frame "叶绿素" {
        }
        frame "藻密度" {
        }
        frame "ORP" {
        }
      }
    }
    frame "i13014" {
      # "稀释倍数"
      n80 = property class="Enum (严格)"(reference=w563) -> ("RingText.Text"=w567:string)  [unwired: 1 in, 2 out]
      n81 = case shown="\"\", 默认" w562 {
        tunnel: [FALSE TRUE TRUE TRUE TRUE TRUE TRUE TRUE TRUE TRUE TRUE TRUE TRUE TRUE] -> w565
        tunnel: [T3 {"status"=TRUE, "代码"=3, "source"=""} ("error out") T3 {"status"=TRUE, "代码"=3, "source"=""} ("error out") T3 {"status"=TRUE, "代码"=3, "source"=""} ("error out") T3 {"status"=TRUE, "代码"=3, "source"=""} ("error out") T3 {"status"=TRUE, "代码"=3, "source"=""} ("error out") T3 {"status"=TRUE, "代码"=3, "source"=""} ("error out") T3 {"status"=TRUE, "代码"=3, "source"=""} ("error out") T3 {"status"=TRUE, "代码"=3, "source"=""} ("error out") T3 {"status"=TRUE, "代码"=3, "source"=""} ("error out") T3 {"status"=TRUE, "代码"=3, "source"=""} ("error out") T3 {"status"=TRUE, "代码"=3, "source"=""} ("error out") T3 {"status"=TRUE, "代码"=3, "source"=""} ("error out") T3 {"status"=TRUE, "代码"=3, "source"=""} ("error out") T3 {"status"=TRUE, "代码"=3, "source"=""} ("error out")] -> w566
        frame "", Default {
        }
        frame "CODMn" {
        }
        frame "PH" {
        }
        frame "氨氮" {
        }
        frame "总氮" {
        }
        frame "总磷" {
        }
        frame "CODCr" {
        }
        frame "电导率" {
        }
        frame "水温" {
        }
        frame "溶解氧" {
        }
        frame "浊度" {
        }
        frame "叶绿素" {
        }
        frame "藻密度" {
        }
        frame "ORP" {
        }
      }
    }
    frame "i13015" {
      # "三项式系数"
      n82 = property class="Enum (严格)"(reference=w597) -> ("RingText.Text"=w601:string)  [unwired: 1 in, 2 out]
      n83 = case shown="\"\", 默认" w596 {
        tunnel: [FALSE TRUE TRUE TRUE TRUE TRUE TRUE TRUE TRUE TRUE TRUE TRUE TRUE TRUE] -> w599
        tunnel: [T3 {"status"=TRUE, "代码"=3, "source"=""} ("error out") T3 {"status"=TRUE, "代码"=3, "source"=""} ("error out") T3 {"status"=TRUE, "代码"=3, "source"=""} ("error out") T3 {"status"=TRUE, "代码"=3, "source"=""} ("error out") T3 {"status"=TRUE, "代码"=3, "source"=""} ("error out") T3 {"status"=TRUE, "代码"=3, "source"=""} ("error out") T3 {"status"=TRUE, "代码"=3, "source"=""} ("error out") T3 {"status"=TRUE, "代码"=3, "source"=""} ("error out") T3 {"status"=TRUE, "代码"=3, "source"=""} ("error out") T3 {"status"=TRUE, "代码"=3, "source"=""} ("error out") T3 {"status"=TRUE, "代码"=3, "source"=""} ("error out") T3 {"status"=TRUE, "代码"=3, "source"=""} ("error out") T3 {"status"=TRUE, "代码"=3, "source"=""} ("error out") T3 {"status"=TRUE, "代码"=3, "source"=""} ("error out")] -> w600
        frame "", Default {
        }
        frame "CODMn" {
        }
        frame "PH" {
        }
        frame "氨氮" {
        }
        frame "总氮" {
        }
        frame "总磷" {
        }
        frame "CODCr" {
        }
        frame "电导率" {
        }
        frame "水温" {
        }
        frame "溶解氧" {
        }
        frame "浊度" {
        }
        frame "叶绿素" {
        }
        frame "藻密度" {
        }
        frame "ORP" {
        }
      }
    }
    frame "i13016" {
      # "空白标定系数"
      n84 = property class="Enum (严格)"(reference=w631) -> ("RingText.Text"=w635:string)  [unwired: 1 in, 2 out]
      n85 = case shown="\"\", 默认" w630 {
        tunnel: [FALSE TRUE TRUE TRUE TRUE TRUE TRUE TRUE TRUE TRUE TRUE TRUE TRUE TRUE] -> w633
        tunnel: [T3 {"status"=TRUE, "代码"=3, "source"=""} ("error out") T3 {"status"=TRUE, "代码"=3, "source"=""} ("error out") T3 {"status"=TRUE, "代码"=3, "source"=""} ("error out") T3 {"status"=TRUE, "代码"=3, "source"=""} ("error out") T3 {"status"=TRUE, "代码"=3, "source"=""} ("error out") T3 {"status"=TRUE, "代码"=3, "source"=""} ("error out") T3 {"status"=TRUE, "代码"=3, "source"=""} ("error out") T3 {"status"=TRUE, "代码"=3, "source"=""} ("error out") T3 {"status"=TRUE, "代码"=3, "source"=""} ("error out") T3 {"status"=TRUE, "代码"=3, "source"=""} ("error out") T3 {"status"=TRUE, "代码"=3, "source"=""} ("error out") T3 {"status"=TRUE, "代码"=3, "source"=""} ("error out") T3 {"status"=TRUE, "代码"=3, "source"=""} ("error out") T3 {"status"=TRUE, "代码"=3, "source"=""} ("error out")] -> w634
        frame "", Default {
        }
        frame "CODMn" {
        }
        frame "PH" {
        }
        frame "氨氮" {
        }
        frame "总氮" {
        }
        frame "总磷" {
        }
        frame "CODCr" {
        }
        frame "电导率" {
        }
        frame "水温" {
        }
        frame "溶解氧" {
        }
        frame "浊度" {
        }
        frame "叶绿素" {
        }
        frame "藻密度" {
        }
        frame "ORP" {
        }
      }
    }
    frame "i13017" {
      # "量程系数"
      n86 = property class="Enum (严格)"(reference=w665) -> ("RingText.Text"=w669:string)  [unwired: 1 in, 2 out]
      n87 = case shown="\"\", 默认" w664 {
        tunnel: [FALSE TRUE TRUE TRUE TRUE TRUE TRUE TRUE TRUE TRUE TRUE TRUE TRUE TRUE] -> w667
        tunnel: [T3 {"status"=TRUE, "代码"=3, "source"=""} ("error out") T3 {"status"=TRUE, "代码"=3, "source"=""} ("error out") T3 {"status"=TRUE, "代码"=3, "source"=""} ("error out") T3 {"status"=TRUE, "代码"=3, "source"=""} ("error out") T3 {"status"=TRUE, "代码"=3, "source"=""} ("error out") T3 {"status"=TRUE, "代码"=3, "source"=""} ("error out") T3 {"status"=TRUE, "代码"=3, "source"=""} ("error out") T3 {"status"=TRUE, "代码"=3, "source"=""} ("error out") T3 {"status"=TRUE, "代码"=3, "source"=""} ("error out") T3 {"status"=TRUE, "代码"=3, "source"=""} ("error out") T3 {"status"=TRUE, "代码"=3, "source"=""} ("error out") T3 {"status"=TRUE, "代码"=3, "source"=""} ("error out") T3 {"status"=TRUE, "代码"=3, "source"=""} ("error out") T3 {"status"=TRUE, "代码"=3, "source"=""} ("error out")] -> w668
        frame "", Default {
        }
        frame "CODMn" {
        }
        frame "PH" {
        }
        frame "氨氮" {
        }
        frame "总氮" {
        }
        frame "总磷" {
        }
        frame "CODCr" {
        }
        frame "电导率" {
        }
        frame "水温" {
        }
        frame "溶解氧" {
        }
        frame "浊度" {
        }
        frame "叶绿素" {
        }
        frame "藻密度" {
        }
        frame "ORP" {
        }
      }
    }
    frame "i13101" {
      # "F0/ORPA"
      n88 = property class="Enum (严格)"(reference=w699) -> ("RingText.Text"=w703:string)  [unwired: 1 in, 2 out]
      n89 = case shown="\"\", 默认" w698 {
        tunnel: [FALSE TRUE TRUE TRUE TRUE TRUE TRUE TRUE TRUE TRUE TRUE TRUE TRUE TRUE] -> w701
        tunnel: [T3 {"status"=TRUE, "代码"=3, "source"=""} ("error out") T3 {"status"=TRUE, "代码"=3, "source"=""} ("error out") T3 {"status"=TRUE, "代码"=3, "source"=""} ("error out") T3 {"status"=TRUE, "代码"=3, "source"=""} ("error out") T3 {"status"=TRUE, "代码"=3, "source"=""} ("error out") T3 {"status"=TRUE, "代码"=3, "source"=""} ("error out") T3 {"status"=TRUE, "代码"=3, "source"=""} ("error out") T3 {"status"=TRUE, "代码"=3, "source"=""} ("error out") T3 {"status"=TRUE, "代码"=3, "source"=""} ("error out") T3 {"status"=TRUE, "代码"=3, "source"=""} ("error out") T3 {"status"=TRUE, "代码"=3, "source"=""} ("error out") T3 {"status"=TRUE, "代码"=3, "source"=""} ("error out") T3 {"status"=TRUE, "代码"=3, "source"=""} ("error out") T3 {"status"=TRUE, "代码"=3, "source"=""} ("error out")] -> w702
        frame "", Default {
        }
        frame "CODMn" {
        }
        frame "PH" {
        }
        frame "氨氮" {
        }
        frame "总氮" {
        }
        frame "总磷" {
        }
        frame "CODCr" {
        }
        frame "电导率" {
        }
        frame "水温" {
        }
        frame "溶解氧" {
        }
        frame "浊度" {
        }
        frame "叶绿素" {
        }
        frame "藻密度" {
        }
        frame "ORP" {
        }
      }
    }
    frame "i13102" {
      # "F1/ORPB"
      n90 = property class="Enum (严格)"(reference=w733) -> ("RingText.Text"=w737:string)  [unwired: 1 in, 2 out]
      n91 = case shown="\"\", 默认" w732 {
        tunnel: [FALSE TRUE TRUE TRUE TRUE TRUE TRUE TRUE TRUE TRUE TRUE TRUE TRUE TRUE] -> w735
        tunnel: [T3 {"status"=TRUE, "代码"=3, "source"=""} ("error out") T3 {"status"=TRUE, "代码"=3, "source"=""} ("error out") T3 {"status"=TRUE, "代码"=3, "source"=""} ("error out") T3 {"status"=TRUE, "代码"=3, "source"=""} ("error out") T3 {"status"=TRUE, "代码"=3, "source"=""} ("error out") T3 {"status"=TRUE, "代码"=3, "source"=""} ("error out") T3 {"status"=TRUE, "代码"=3, "source"=""} ("error out") T3 {"status"=TRUE, "代码"=3, "source"=""} ("error out") T3 {"status"=TRUE, "代码"=3, "source"=""} ("error out") T3 {"status"=TRUE, "代码"=3, "source"=""} ("error out") T3 {"status"=TRUE, "代码"=3, "source"=""} ("error out") T3 {"status"=TRUE, "代码"=3, "source"=""} ("error out") T3 {"status"=TRUE, "代码"=3, "source"=""} ("error out") T3 {"status"=TRUE, "代码"=3, "source"=""} ("error out")] -> w736
        frame "", Default {
        }
        frame "CODMn" {
        }
        frame "PH" {
        }
        frame "氨氮" {
        }
        frame "总氮" {
        }
        frame "总磷" {
        }
        frame "CODCr" {
        }
        frame "电导率" {
        }
        frame "水温" {
        }
        frame "溶解氧" {
        }
        frame "浊度" {
        }
        frame "叶绿素" {
        }
        frame "藻密度" {
        }
        frame "ORP" {
        }
      }
    }
    frame "i13103" {
      # "F2/ORPK"
      n92 = property class="Enum (严格)"(reference=w767) -> ("RingText.Text"=w771:string)  [unwired: 1 in, 2 out]
      n93 = case shown="\"\", 默认" w766 {
        tunnel: [FALSE TRUE TRUE TRUE TRUE TRUE TRUE TRUE TRUE TRUE TRUE TRUE TRUE TRUE] -> w769
        tunnel: [T3 {"status"=TRUE, "代码"=3, "source"=""} ("error out") T3 {"status"=TRUE, "代码"=3, "source"=""} ("error out") T3 {"status"=TRUE, "代码"=3, "source"=""} ("error out") T3 {"status"=TRUE, "代码"=3, "source"=""} ("error out") T3 {"status"=TRUE, "代码"=3, "source"=""} ("error out") T3 {"status"=TRUE, "代码"=3, "source"=""} ("error out") T3 {"status"=TRUE, "代码"=3, "source"=""} ("error out") T3 {"status"=TRUE, "代码"=3, "source"=""} ("error out") T3 {"status"=TRUE, "代码"=3, "source"=""} ("error out") T3 {"status"=TRUE, "代码"=3, "source"=""} ("error out") T3 {"status"=TRUE, "代码"=3, "source"=""} ("error out") T3 {"status"=TRUE, "代码"=3, "source"=""} ("error out") T3 {"status"=TRUE, "代码"=3, "source"=""} ("error out") T3 {"status"=TRUE, "代码"=3, "source"=""} ("error out")] -> w770
        frame "", Default {
        }
        frame "CODMn" {
        }
        frame "PH" {
        }
        frame "氨氮" {
        }
        frame "总氮" {
        }
        frame "总磷" {
        }
        frame "CODCr" {
        }
        frame "电导率" {
        }
        frame "水温" {
        }
        frame "溶解氧" {
        }
        frame "浊度" {
        }
        frame "叶绿素" {
        }
        frame "藻密度" {
        }
        frame "ORP" {
        }
      }
    }
    frame "i13104" {
      # "F3"
      n94 = property class="Enum (严格)"(reference=w805) -> ("RingText.Text"=w803:string)  [unwired: 1 in, 2 out]
      n95 = case shown="\"\", 默认" w804 {
        tunnel: [FALSE TRUE TRUE TRUE TRUE TRUE TRUE TRUE TRUE TRUE TRUE TRUE TRUE TRUE] -> w801
        tunnel: [T3 {"status"=TRUE, "代码"=3, "source"=""} ("error out") T3 {"status"=TRUE, "代码"=3, "source"=""} ("error out") T3 {"status"=TRUE, "代码"=3, "source"=""} ("error out") T3 {"status"=TRUE, "代码"=3, "source"=""} ("error out") T3 {"status"=TRUE, "代码"=3, "source"=""} ("error out") T3 {"status"=TRUE, "代码"=3, "source"=""} ("error out") T3 {"status"=TRUE, "代码"=3, "source"=""} ("error out") T3 {"status"=TRUE, "代码"=3, "source"=""} ("error out") T3 {"status"=TRUE, "代码"=3, "source"=""} ("error out") T3 {"status"=TRUE, "代码"=3, "source"=""} ("error out") T3 {"status"=TRUE, "代码"=3, "source"=""} ("error out") T3 {"status"=TRUE, "代码"=3, "source"=""} ("error out") T3 {"status"=TRUE, "代码"=3, "source"=""} ("error out") T3 {"status"=TRUE, "代码"=3, "source"=""} ("error out")] -> w802
        frame "", Default {
        }
        frame "CODMn" {
        }
        frame "PH" {
        }
        frame "氨氮" {
        }
        frame "总氮" {
        }
        frame "总磷" {
        }
        frame "CODCr" {
        }
        frame "电导率" {
        }
        frame "水温" {
        }
        frame "溶解氧" {
        }
        frame "浊度" {
        }
        frame "叶绿素" {
        }
        frame "藻密度" {
        }
        frame "ORP" {
        }
      }
    }
    frame "i13105" {
      # "F4"
      n96 = property class="Enum (严格)"(reference=w835) -> ("RingText.Text"=w839:string)  [unwired: 1 in, 2 out]
      n97 = case shown="\"\", 默认" w834 {
        tunnel: [FALSE TRUE TRUE TRUE TRUE TRUE TRUE TRUE TRUE TRUE TRUE TRUE TRUE TRUE] -> w837
        tunnel: [T3 {"status"=TRUE, "代码"=3, "source"=""} ("error out") T3 {"status"=TRUE, "代码"=3, "source"=""} ("error out") T3 {"status"=TRUE, "代码"=3, "source"=""} ("error out") T3 {"status"=TRUE, "代码"=3, "source"=""} ("error out") T3 {"status"=TRUE, "代码"=3, "source"=""} ("error out") T3 {"status"=TRUE, "代码"=3, "source"=""} ("error out") T3 {"status"=TRUE, "代码"=3, "source"=""} ("error out") T3 {"status"=TRUE, "代码"=3, "source"=""} ("error out") T3 {"status"=TRUE, "代码"=3, "source"=""} ("error out") T3 {"status"=TRUE, "代码"=3, "source"=""} ("error out") T3 {"status"=TRUE, "代码"=3, "source"=""} ("error out") T3 {"status"=TRUE, "代码"=3, "source"=""} ("error out") T3 {"status"=TRUE, "代码"=3, "source"=""} ("error out") T3 {"status"=TRUE, "代码"=3, "source"=""} ("error out")] -> w838
        frame "", Default {
        }
        frame "CODMn" {
        }
        frame "PH" {
        }
        frame "氨氮" {
        }
        frame "总氮" {
        }
        frame "总磷" {
        }
        frame "CODCr" {
        }
        frame "电导率" {
        }
        frame "水温" {
        }
        frame "溶解氧" {
        }
        frame "浊度" {
        }
        frame "叶绿素" {
        }
        frame "藻密度" {
        }
        frame "ORP" {
        }
      }
    }
    frame "i13106" {
      # "F5"
      n98 = property class="Enum (严格)"(reference=w869) -> ("RingText.Text"=w873:string)  [unwired: 1 in, 2 out]
      n99 = case shown="\"\", 默认" w868 {
        tunnel: [FALSE TRUE TRUE TRUE TRUE TRUE TRUE TRUE TRUE TRUE TRUE TRUE TRUE TRUE] -> w871
        tunnel: [T3 {"status"=TRUE, "代码"=3, "source"=""} ("error out") T3 {"status"=TRUE, "代码"=3, "source"=""} ("error out") T3 {"status"=TRUE, "代码"=3, "source"=""} ("error out") T3 {"status"=TRUE, "代码"=3, "source"=""} ("error out") T3 {"status"=TRUE, "代码"=3, "source"=""} ("error out") T3 {"status"=TRUE, "代码"=3, "source"=""} ("error out") T3 {"status"=TRUE, "代码"=3, "source"=""} ("error out") T3 {"status"=TRUE, "代码"=3, "source"=""} ("error out") T3 {"status"=TRUE, "代码"=3, "source"=""} ("error out") T3 {"status"=TRUE, "代码"=3, "source"=""} ("error out") T3 {"status"=TRUE, "代码"=3, "source"=""} ("error out") T3 {"status"=TRUE, "代码"=3, "source"=""} ("error out") T3 {"status"=TRUE, "代码"=3, "source"=""} ("error out") T3 {"status"=TRUE, "代码"=3, "source"=""} ("error out")] -> w872
        frame "", Default {
        }
        frame "CODMn" {
        }
        frame "PH" {
        }
        frame "氨氮" {
        }
        frame "总氮" {
        }
        frame "总磷" {
        }
        frame "CODCr" {
        }
        frame "电导率" {
        }
        frame "水温" {
        }
        frame "溶解氧" {
        }
        frame "浊度" {
        }
        frame "叶绿素" {
        }
        frame "藻密度" {
        }
        frame "ORP" {
        }
      }
    }
    frame "i13107" {
      # "F6"
      n100 = property class="Enum (严格)"(reference=w903) -> ("RingText.Text"=w907:string)  [unwired: 1 in, 2 out]
      n101 = case shown="\"\", 默认" w902 {
        tunnel: [FALSE TRUE TRUE TRUE TRUE TRUE TRUE TRUE TRUE TRUE TRUE TRUE TRUE TRUE] -> w905
        tunnel: [T3 {"status"=TRUE, "代码"=3, "source"=""} ("error out") T3 {"status"=TRUE, "代码"=3, "source"=""} ("error out") T3 {"status"=TRUE, "代码"=3, "source"=""} ("error out") T3 {"status"=TRUE, "代码"=3, "source"=""} ("error out") T3 {"status"=TRUE, "代码"=3, "source"=""} ("error out") T3 {"status"=TRUE, "代码"=3, "source"=""} ("error out") T3 {"status"=TRUE, "代码"=3, "source"=""} ("error out") T3 {"status"=TRUE, "代码"=3, "source"=""} ("error out") T3 {"status"=TRUE, "代码"=3, "source"=""} ("error out") T3 {"status"=TRUE, "代码"=3, "source"=""} ("error out") T3 {"status"=TRUE, "代码"=3, "source"=""} ("error out") T3 {"status"=TRUE, "代码"=3, "source"=""} ("error out") T3 {"status"=TRUE, "代码"=3, "source"=""} ("error out") T3 {"status"=TRUE, "代码"=3, "source"=""} ("error out")] -> w906
        frame "", Default {
        }
        frame "CODMn" {
        }
        frame "PH" {
        }
        frame "氨氮" {
        }
        frame "总氮" {
        }
        frame "总磷" {
        }
        frame "CODCr" {
        }
        frame "电导率" {
        }
        frame "水温" {
        }
        frame "溶解氧" {
        }
        frame "浊度" {
        }
        frame "叶绿素" {
        }
        frame "藻密度" {
        }
        frame "ORP" {
        }
      }
    }
    frame "i13108" {
      # "F7"
      n102 = property class="Enum (严格)"(reference=w937) -> ("RingText.Text"=w941:string)  [unwired: 1 in, 2 out]
      n103 = case shown="\"\", 默认" w936 {
        tunnel: [FALSE TRUE TRUE TRUE TRUE TRUE TRUE TRUE TRUE TRUE TRUE TRUE TRUE TRUE] -> w939
        tunnel: [T3 {"status"=TRUE, "代码"=3, "source"=""} ("error out") T3 {"status"=TRUE, "代码"=3, "source"=""} ("error out") T3 {"status"=TRUE, "代码"=3, "source"=""} ("error out") T3 {"status"=TRUE, "代码"=3, "source"=""} ("error out") T3 {"status"=TRUE, "代码"=3, "source"=""} ("error out") T3 {"status"=TRUE, "代码"=3, "source"=""} ("error out") T3 {"status"=TRUE, "代码"=3, "source"=""} ("error out") T3 {"status"=TRUE, "代码"=3, "source"=""} ("error out") T3 {"status"=TRUE, "代码"=3, "source"=""} ("error out") T3 {"status"=TRUE, "代码"=3, "source"=""} ("error out") T3 {"status"=TRUE, "代码"=3, "source"=""} ("error out") T3 {"status"=TRUE, "代码"=3, "source"=""} ("error out") T3 {"status"=TRUE, "代码"=3, "source"=""} ("error out") T3 {"status"=TRUE, "代码"=3, "source"=""} ("error out")] -> w940
        frame "", Default {
        }
        frame "CODMn" {
        }
        frame "PH" {
        }
        frame "氨氮" {
        }
        frame "总氮" {
        }
        frame "总磷" {
        }
        frame "CODCr" {
        }
        frame "电导率" {
        }
        frame "水温" {
        }
        frame "溶解氧" {
        }
        frame "浊度" {
        }
        frame "叶绿素" {
        }
        frame "藻密度" {
        }
        frame "ORP" {
        }
      }
    }
    frame "i13109" {
      # "X0/滴定数"
      n104 = property class="Enum (严格)"(reference=w971) -> ("RingText.Text"=w975:string)  [unwired: 1 in, 2 out]
      n105 = case shown="\"\", 默认" w970 {
        tunnel: [FALSE TRUE TRUE TRUE TRUE TRUE TRUE TRUE TRUE TRUE TRUE TRUE TRUE TRUE] -> w973
        tunnel: [T3 {"status"=TRUE, "代码"=3, "source"=""} ("error out") T3 {"status"=TRUE, "代码"=3, "source"=""} ("error out") T3 {"status"=TRUE, "代码"=3, "source"=""} ("error out") T3 {"status"=TRUE, "代码"=3, "source"=""} ("error out") T3 {"status"=TRUE, "代码"=3, "source"=""} ("error out") T3 {"status"=TRUE, "代码"=3, "source"=""} ("error out") T3 {"status"=TRUE, "代码"=3, "source"=""} ("error out") T3 {"status"=TRUE, "代码"=3, "source"=""} ("error out") T3 {"status"=TRUE, "代码"=3, "source"=""} ("error out") T3 {"status"=TRUE, "代码"=3, "source"=""} ("error out") T3 {"status"=TRUE, "代码"=3, "source"=""} ("error out") T3 {"status"=TRUE, "代码"=3, "source"=""} ("error out") T3 {"status"=TRUE, "代码"=3, "source"=""} ("error out") T3 {"status"=TRUE, "代码"=3, "source"=""} ("error out")] -> w974
        frame "", Default {
        }
        frame "CODMn" {
        }
        frame "PH" {
        }
        frame "氨氮" {
        }
        frame "总氮" {
        }
        frame "总磷" {
        }
        frame "CODCr" {
        }
        frame "电导率" {
        }
        frame "水温" {
        }
        frame "溶解氧" {
        }
        frame "浊度" {
        }
        frame "叶绿素" {
        }
        frame "藻密度" {
        }
        frame "ORP" {
        }
      }
    }
    frame "i13110" {
      # "量程"
      n106 = property class="Enum (严格)"(reference=w1005) -> ("RingText.Text"=w1009:string)  [unwired: 1 in, 2 out]
      n107 = case shown="\"\", 默认" w1004 {
        tunnel: [FALSE TRUE TRUE TRUE TRUE TRUE TRUE TRUE TRUE TRUE TRUE TRUE TRUE TRUE] -> w1007
        tunnel: [T3 {"status"=TRUE, "代码"=3, "source"=""} ("error out") T3 {"status"=TRUE, "代码"=3, "source"=""} ("error out") T3 {"status"=TRUE, "代码"=3, "source"=""} ("error out") T3 {"status"=TRUE, "代码"=3, "source"=""} ("error out") T3 {"status"=TRUE, "代码"=3, "source"=""} ("error out") T3 {"status"=TRUE, "代码"=3, "source"=""} ("error out") T3 {"status"=TRUE, "代码"=3, "source"=""} ("error out") T3 {"status"=TRUE, "代码"=3, "source"=""} ("error out") T3 {"status"=TRUE, "代码"=3, "source"=""} ("error out") T3 {"status"=TRUE, "代码"=3, "source"=""} ("error out") T3 {"status"=TRUE, "代码"=3, "source"=""} ("error out") T3 {"status"=TRUE, "代码"=3, "source"=""} ("error out") T3 {"status"=TRUE, "代码"=3, "source"=""} ("error out") T3 {"status"=TRUE, "代码"=3, "source"=""} ("error out")] -> w1008
        frame "", Default {
        }
        frame "CODMn" {
        }
        frame "PH" {
        }
        frame "氨氮" {
        }
        frame "总氮" {
        }
        frame "总磷" {
        }
        frame "CODCr" {
        }
        frame "电导率" {
        }
        frame "水温" {
        }
        frame "溶解氧" {
        }
        frame "浊度" {
        }
        frame "叶绿素" {
        }
        frame "藻密度" {
        }
        frame "ORP" {
        }
      }
    }
  }
  n108 = case shown="真" w8 {
    tunnel: w6 -> [_ w1040]
    tunnel: w5 -> [_ w1039]
    tunnel: w4 -> [_ w1038]
    frame False {
    }
    frame True {
      n109 = call "执行结果反馈与日志存储.vi"("日志信息"=w1039, "error out"=w1038, "设备"=w1040) -> ()  [unwired: 9 in]
    }
  }
